vi "SetProjectorParameters.vi"(0 "PowerLevel (High Normal Low)":u8(ring) items=["High", "Normal", "Low"], 1 "FringeCodingMode (Fast Accurate Translucent Reflective)":u8(ring) items=["Fast", "Accurate", "Translucent", "Reflective"], 4 "AntiFlickerMode (Off AC50Hz AC60Hz)":u8(ring) items=["Off", "AC50Hz", "AC60Hz"], 5 "error in (no error)":errorcluster, 6 "Camera Reference in":refnum<k24>) -> (2 "error out":errorcluster, 3 "Camera Reference out":refnum<k24>)   [LabVIEW 2023]
uses:
  C:/Mech-Mind/Mech-Eye SDK-2.5.0-b5-dev-01-03/API/dll/net48/MechEyeApiNet.dll
  dll/net48/MechEyeApiNet.dll
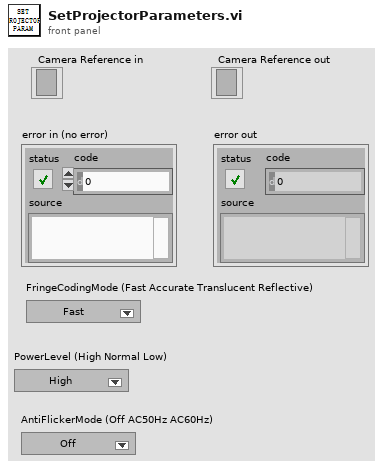
[diagram p1: front panel]
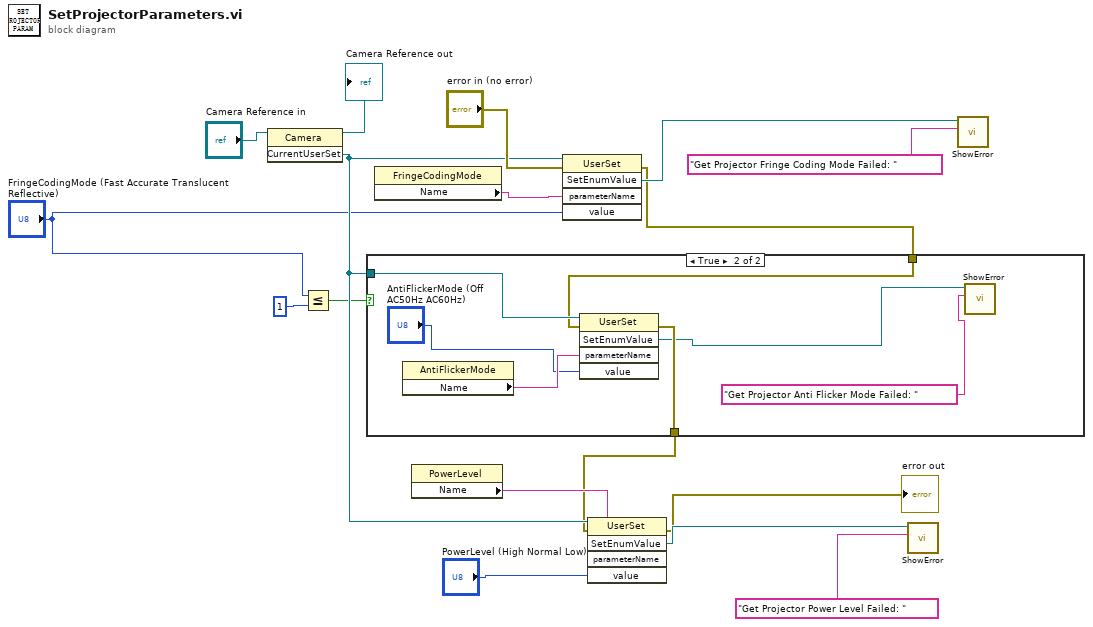
[diagram p0: block diagram]
diagram:
  n1 = invoke class="Camera" method="CurrentUserSet"(reference="Camera Reference in") -> (reference out=→"Camera Reference out":refnum<k24>, "CurrentUserSet"=w6:refnum<k24>)  [unwired: 2 in, 1 out]
  n2 = Less Or Equal?(x="FringeCodingMode (Fast Accurate Translucent Reflective)", y=1) -> (x <= y?=w1:bool)
  n3 = property class="FringeCodingMode"() -> ("Name"=w14:string)  [unwired: 2 in, 2 out]
  n4 = property class="PowerLevel"() -> ("Name"=w12:string)  [unwired: 2 in, 2 out]
  n5 = invoke class="UserSet" method="SetEnumValue"(reference=w6, error in="error in (no error)", "parameterName"=w14, "value"="FringeCodingMode (Fast Accurate Translucent Reflective)") -> (error out=w5:errorcluster, "SetEnumValue"=w13:refnum<k24>)  [unwired: 1 in, 3 out]
  n6 = case shown="True" w1 {
    tunnel: w6 -> [_ w25]
    tunnel: w5 -> [w18 w24]
    tunnel: [w18 w21] -> w4
    frame False {
    }
    frame True {
      n7 = property class="AntiFlickerMode"() -> ("Name"=w23:string)  [unwired: 2 in, 2 out]
      n8 = invoke class="UserSet" method="SetEnumValue"(reference=w25, error in=w24, "parameterName"=w23, "value"="AntiFlickerMode (Off AC50Hz AC60Hz)") -> (error out=w21:errorcluster, "SetEnumValue"=w19:refnum<k24>)  [unwired: 1 in, 3 out]
      n9 = call "ShowError.vi"("String"="Get Projector Anti Flicker Mode Failed: ", "MMind.Eye.ErrorStatus"=w19) -> ()  [unwired: 10 in]
    }
  }
  n10 = invoke class="UserSet" method="SetEnumValue"(reference=w6, error in=w4, "parameterName"=w12, "value"="PowerLevel (High Normal Low)") -> (error out=→"error out":errorcluster, "SetEnumValue"=w11:refnum<k24>)  [unwired: 1 in, 3 out]
  n11 = call "ShowError.vi"("String"="Get Projector Power Level Failed: ", "MMind.Eye.ErrorStatus"=w11) -> ()  [unwired: 10 in]
  n12 = call "ShowError.vi"("String"="Get Projector Fringe Coding Mode Failed: ", "MMind.Eye.ErrorStatus"=w13) -> ()  [unwired: 10 in]
